vi "test Add State.vi"(8 "error in (no error)":errorcluster, 11 "TestCase in":refnum<class "Routing and Faulting State Value Table Unit Tests.lvclass">) -> (0 "error out":errorcluster, 3 "TestCase out":refnum<class "Routing and Faulting State Value Table Unit Tests.lvclass">)   [LabVIEW 2020, in "Routing and Faulting State Value Table Unit Tests.lvclass"]
uses:
  Routing and Faulting State Value Table Unit Tests.lvclass
  System Explorer/State-Value Row.ctl
  Shared/Channel States.ctl
  Shared/Routing State.ctl
  Shared/Connection.ctl
  Routing and Faulting State Value Table Unit Tests.lvclass/Routing and Faulting State Value Table Unit Tests.ctl
  <vilib>/addons/_JKI Toolkits/VI Tester/TestCase.llb/TestCase.lvclass
  System Explorer/Routing and Faulting System Explorer.lvlib
  Shared/Routing and Faulting Shared.lvlib
  Scripting/Routing and Faulting Scripting.lvlib
  C:/Program Files (x86)/National Instruments/LabVIEW 2020/vi.lib/addons/_JKI Toolkits/VI Tester/TestCase.llb/TestCase.lvclass
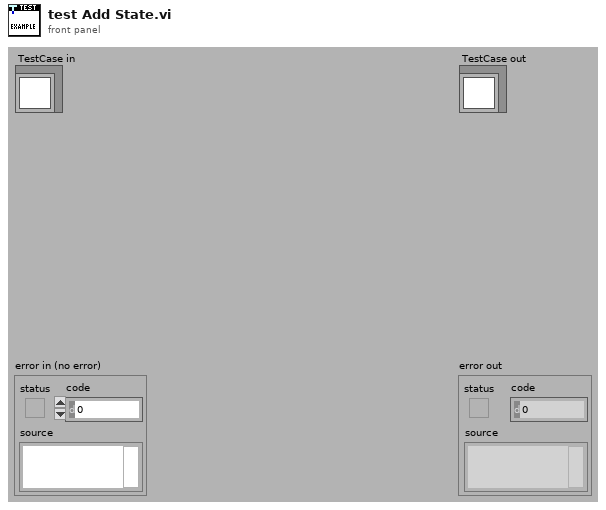
[diagram p1: front panel]
types:
  T1 = typedef "Routing and Faulting System Explorer.lvlib/State-Value Row.ctl" = cluster{"State":string, "State Value":string}
  T2 = typedef "Routing and Faulting Shared.lvlib/Channel States.ctl" = T3[]
  T3 = typedef "Routing and Faulting Shared.lvlib/Routing State.ctl" = cluster{"Name":string, "Description":string, "Value":i32, "Connection List":T4[]}
  T4 = typedef "Routing and Faulting Shared.lvlib/Connection.ctl" = cluster{"Module":string, "Source":string, "Destination":string}
  T5 = typedef "Custom Device API.lvlib/Custom Device Item Ref.ctl" = u64
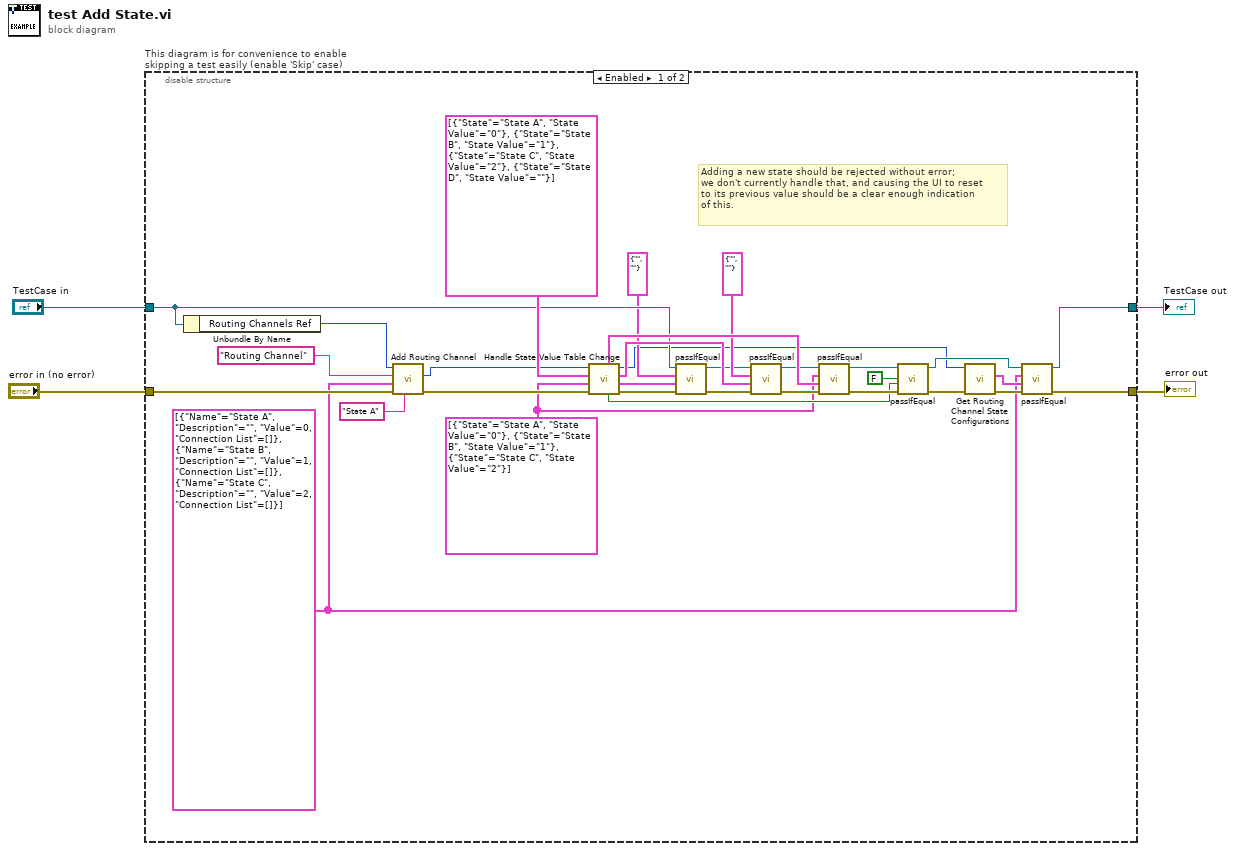
[diagram p0: block diagram]
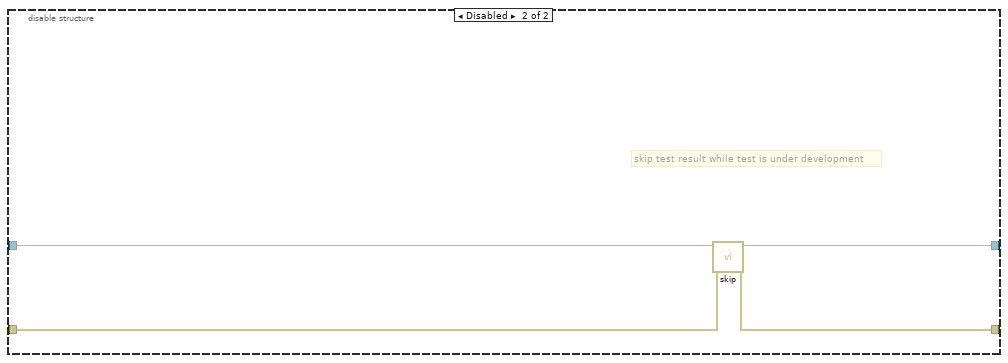
[diagram p2: hidden frame]
diagram:
  n1 = disable-structure "This diagram is for convenience to enable skipping a test easily (enable 'Skip' case)" shown="Enabled" {
    disable-tunnel: "TestCase in" -> [w20 w39]
    disable-tunnel: [w10 w37] -> w1
    disable-tunnel: [w11 w38] -> w3
    disable-tunnel: "error in (no error)" -> [w35 w36]
    frame Enabled {
      w6 = T1[] [{"State"="State A", "State Value"="0"}, {"State"="State B", "State Value"="1"}, {"State"="State C", "State Value"="2"}] ("NewVal")
      w5 = T2 [{"Name"="State A", "Description"="", "Value"=0, "Connection List"=[]}, {"Name"="State B", "Description"="", "Value"=1, "Connection List"=[]}, {"Name"="State C", "Description"="", "Value"=2, "Connection List"=[]}] ("state configurations")
      # "Adding a new state should be rejected without error;\nwe don't currently handle that, and causing the UI to reset\nto its previous value should be a clear enough indication\nof this."
      n2 = Unbundle By Name(w20) -> ("Routing Channels Ref"=w33:T5)
      n3 = call "Add Routing Channel.vi"("initial state"="State A", "error in"=w35, "state configurations"=w5, "channel name"="Routing Channel", "routing channels in"=w33) -> ("error out"=w34:errorcluster, "routing channel"=w27:T5)  [unwired: 4 in, 1 out]
      n4 = call "Handle State Value Table Change.vi"("error in (no error)"=w34, "OldVal"=w6, "NewVal"=T1[] [{"State"="State A", "State Value"="0"}, {"State"="State B", "State Value"="1"}, {"State"="State C", "State Value"="2"}, {"State"="State D", "State Value"=""}], "routing channel in"=w27) -> ("error out"=w17:errorcluster, "old modified state and value"=w21:T1, "new modified state and value"=w24:T1, "routing channel out"=w7:T5, "update controls"=w15:bool, "coerced newval"=w31:T1[])  [unwired: 2 in]
      n5 = call-dynamic "passIfEqual.vi"("error in (no error)"=w17, "y"=w21, "x"=T1 {"State"="", "State Value"=""} ("old modified state and value"), "TestCase in"=w20) -> ("error out"=w22:errorcluster, "TestCase out"=w19:refnum<class "Routing and Faulting State Value Table Unit Tests.lvclass">)  [unwired: 6 in]
      n6 = call-dynamic "passIfEqual.vi"("error in (no error)"=w22, "y"=w24, "x"=T1 {"State"="", "State Value"=""} ("new modified state and value"), "TestCase in"=w19) -> ("error out"=w26:errorcluster, "TestCase out"=w25:refnum<class "Routing and Faulting State Value Table Unit Tests.lvclass">)  [unwired: 6 in]
      n7 = call-dynamic "passIfEqual.vi"("error in (no error)"=w26, "y"=w31, "x"=w6, "TestCase in"=w25) -> ("error out"=w32:errorcluster, "TestCase out"=w16:refnum<class "Routing and Faulting State Value Table Unit Tests.lvclass">)  [unwired: 6 in]
      n8 = call-dynamic "passIfEqual.vi"("error in (no error)"=w32, "y"=w15, "x"=FALSE ("update controls"), "TestCase in"=w16) -> ("error out"=w8:errorcluster, "TestCase out"=w9:refnum<class "Routing and Faulting State Value Table Unit Tests.lvclass">)  [unwired: 6 in]
      n9 = call "Get Routing Channel State Configurations.vi"("error in"=w8, "routing channel in"=w7) -> ("error out"=w13:errorcluster, "state configurations"=w12:T2)  [unwired: 7 in, 1 out]
      n10 = call-dynamic "passIfEqual.vi"("error in (no error)"=w13, "y"=w12, "x"=w5, "TestCase in"=w9) -> ("error out"=w11:errorcluster, "TestCase out"=w10:refnum<class "Routing and Faulting State Value Table Unit Tests.lvclass">)  [unwired: 6 in]
    }
    frame Disabled {
      # "skip test result while test is under development"
      n11 = call <vilib>:"skip.vi"("error in (no error)"=w36, "TestCase in"=w39) -> ("error out"=w38:errorcluster, "TestCase out"=w37:refnum<class "Routing and Faulting State Value Table Unit Tests.lvclass">)  [unwired: 8 in]
    }
  }
  "error out" <- w3
  "TestCase out" <- w1
